vi "ReadDigitalOutput.vi"(8 "error in (no error)":errorcluster, 11 "DigitalOutput_Simulation In":refnum<class "TesteractHAL_DigitalOutput_Simulation.lvclass">) -> (0 "error out":errorcluster, 1 "Tristate":bool, 2 "data":bool, 3 "DigitalOutput_Simulation Out":refnum<class "TesteractHAL_DigitalOutput_Simulation.lvclass">)   [LabVIEW 2017, in "TesteractHAL_DigitalOutput_Simulation.lvlib" / "TesteractHAL_DigitalOutput_Simulation.lvclass"]
doc: "Read a single digital bool."
uses:
  TesteractHAL_DigitalOutput_Simulation.lvclass
  TesteractHAL_DigitalOutput_Simulation.lvclass/TesteractHAL_DigitalOutput_Simulation.ctl
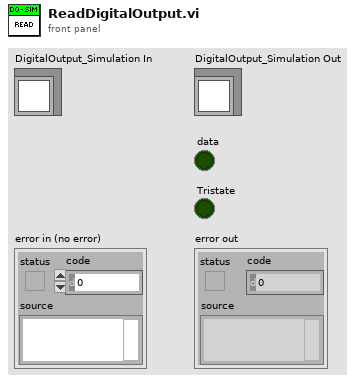
[diagram p1: front panel]
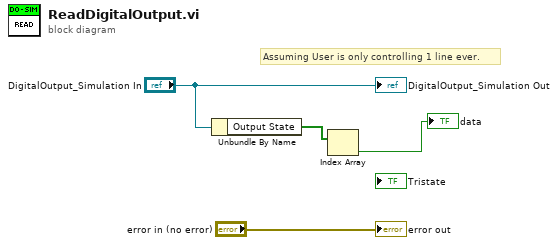
[diagram p0: block diagram]
diagram:
  # "Assuming User is only controlling 1 line ever."
  n1 = Unbundle By Name("DigitalOutput_Simulation In") -> ("Output State"=w2:bool[])
  n2 = Index Array(array=w2) -> (element=→"data":bool)  [unwired: 1 in]
  "error out" <- "error in (no error)"
  "DigitalOutput_Simulation Out" <- "DigitalOutput_Simulation In"
